vi "read a line csv.vi"(8 "에러 입력":errorcluster, 10 "오프셋(바이트) (0)":i64, 11 "참조 번호":refnum<file>) -> (0 "error out":errorcluster, 1 "문자열":string, 2 "last offset":i64, 3 "refnum out":refnum<file>)   [LabVIEW 2015]
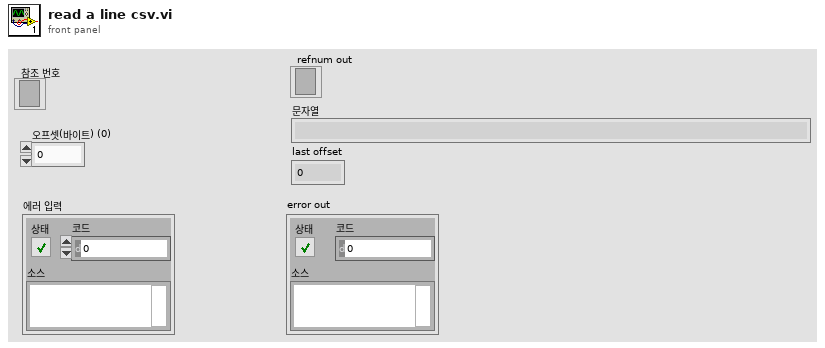
[diagram p1: front panel]
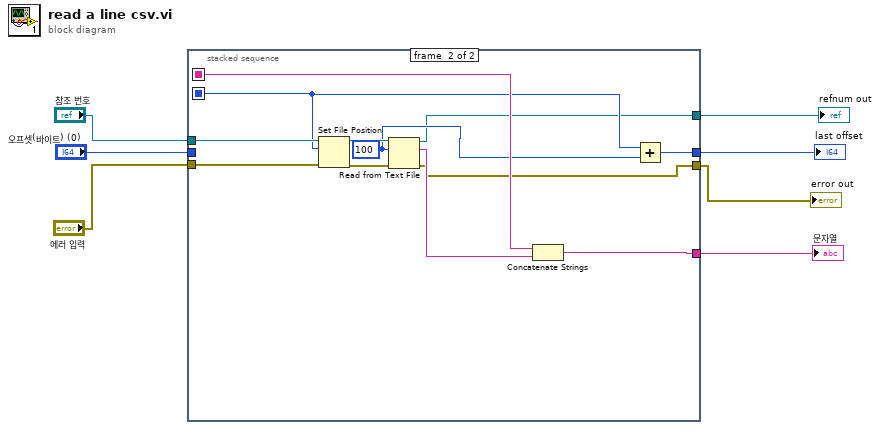
[diagram p0: block diagram]
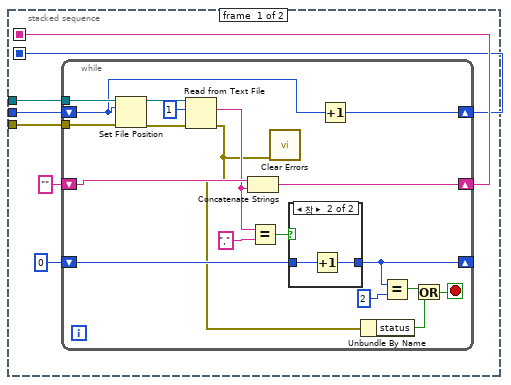
[diagram p2: hidden frame]
diagram:
  n1 = stacked-sequence {
    seq-local: [w9 _] -> [_ w44]
    seq-local: [w8 _] -> [_ w40]
    tunnel: "참조 번호" -> [w14 w46]
    tunnel: "에러 입력" -> [w13 w45]
    tunnel: [_ w38] -> w5
    tunnel: [_ w37] -> w4
    tunnel: [_ w42] -> w3
    tunnel: [_ w41] -> w2
    tunnel: "오프셋(바이트) (0)" -> [w12 _]
    frame #0 {
      n2 = while {
        tunnel: w14 -> [w33]
        tunnel: w13 -> [w32]
        shift-right: [w28] -> w8
        shift-left: w12 -> [w27]
        shift-right: [w26] -> w9
        shift-left: "" -> [w25]
        shift-right: [w20] -> _
        shift-left: 0 -> [w21]
        stop <- w18 stop-if-true
        n3 = Set File Position(offset (in bytes) (0)=w27, refnum=w33, error in=w32) -> (refnum out=w31:refnum<file>, error out=w30:errorcluster)  [unwired: 1 in]
        n4 = Read from Text File(file (use dialog)=w31, count=1 ("카운트"), error in=w30) -> (text=w23:string, error out=w15:errorcluster)  [unwired: 1 in, 2 out]
        n5 = Concatenate Strings(w25, w23) -> (w26:string)
        n6 = Equal?(x=w23, y=",") -> (x = y?=w22:bool)
        n7 = call <vilib>:"Clear Errors.vi"("error in (no error)"=w15) -> ()  [unwired: 5 in, 2 out]
        n8 = case shown="참" w22 {
          tunnel: w21 -> [w34 w36]
          tunnel: [w34 w35] -> w20
          frame False {
          }
          frame True {
            n9 = Increment(x=w36) -> (x+1=w35:i32)
          }
        }
        n10 = Increment(x=w27) -> (x+1=w28:i64)
        n11 = Unbundle By Name(w15) -> ("status"=w16:bool)
        n12 = Equal?(x=w20, y=2) -> (x = y?=w17:bool)
        n13 = Or(x=w17, y=w16) -> (x .or. y?=w18:bool)
      }
    }
    frame #1 {
      w39 = 100 ("카운트")
      n14 = Set File Position(offset (in bytes) (0)=w40, refnum=w46, error in=w45) -> (refnum out=w48:refnum<file>, error out=w47:errorcluster)  [unwired: 1 in]
      n15 = Read from Text File(file (use dialog)=w48, count=w39, error in=w47) -> (refnum out=w37:refnum<file>, text=w43:string, error out=w38:errorcluster)  [unwired: 1 in, 1 out]
      n16 = Concatenate Strings(w44, w43) -> (w42:string)
      n17 = Add(x=w40, y=w39) -> (x+y=w41:i64)
    }
  }
  "문자열" <- w3
  "last offset" <- w2
  "error out" <- w5
  "refnum out" <- w4
